vi "telemetryElevationData.vi"(8 "error in (no error)":errorcluster, 11 "Publisher in":refnum<class "Publisher.lvclass">) -> (0 "error out":errorcluster, 3 "Publisher out":refnum<class "Publisher.lvclass">)   [LabVIEW 2016, in "Publisher.lvclass"]
uses:
  Publisher.lvclass
  Publisher.lvclass/Publisher.ctl
  Communicator/M1M3SAL/M1M3SAL.lvclass/M1M3SAL.ctl
  Communicator/M1M3SAL/writeHeader.vi
  Communicator/M1M3SAL/writeDBL.vi
  Communicator/M1M3SAL/writeU8.vi
  Communicator/M1M3SAL/writeI32.vi
  Communicator/M1M3SAL/M1M3SAL.lvclass
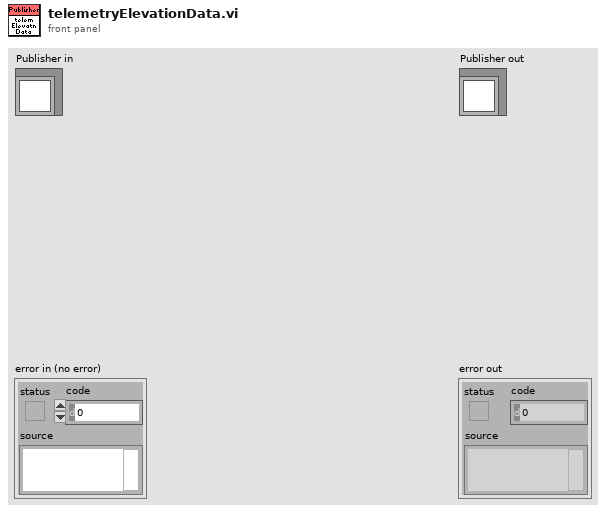
[diagram p1: front panel]
types:
  T1 = typedef "M1M3SupportTopics.lvlib/TelemetryElevationData.ctl" = cluster{"Timestamp":T2, "InclinometerElevation":dbl, "MeasuredElevation":dbl}
  T2 = typedef "M1M3SupportTopics.lvlib/Timestamp.ctl" = dbl
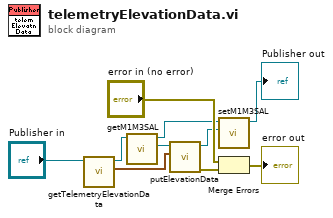
[diagram p0: block diagram]
diagram:
  n1 = call "getTelemetryElevationData.vi"("Publisher in"="Publisher in") -> ("TelemetryElevationData"=w2:T1, "Publisher out"=w6:refnum<class "Publisher.lvclass">)  [unwired: 9 in]
  n2 = call "getM1M3SAL.vi"("Publisher in"=w6) -> ("M1M3SAL"=w3:refnum<class "M1M3SAL.lvclass">, "Publisher out"=w7:refnum<class "Publisher.lvclass">)  [unwired: 9 in]
  n3 = call "putElevationData.vi"("TelemetryElevationData"=w2, "M1M3SAL in"=w3) -> ("error out"=w1:errorcluster, "M1M3SAL out"=w4:refnum<class "M1M3SAL.lvclass">)  [unwired: 8 in]
  n4 = call "setM1M3SAL.vi"("M1M3SAL"=w4, "Publisher in"=w7) -> ("Publisher out"=→"Publisher out":refnum<class "Publisher.lvclass">)  [unwired: 9 in]
  n5 = Merge Errors("error in (no error)", w1) -> (→"error out":errorcluster)
